vi "CloseDevice.vi"(8 "错误输入（无错误）":errorcluster, 11 "DevIndex":i32) -> (0 "错误输出":errorcluster, 3 "DevIndex Output":i32)   [LabVIEW 2018]
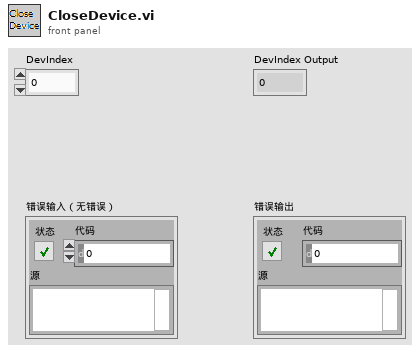
[diagram p1: front panel]
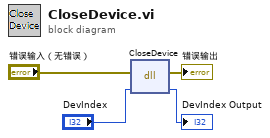
[diagram p0: block diagram]
diagram:
  n1 = dll-call lib="PTH2@abs H科研项目仅一项目程序32位usb-1000.dll" fn="CloseDevice"(error in="错误输入（无错误）", "DevIndex"="DevIndex") -> (error out=→"错误输出":errorcluster, "DevIndex"=→"DevIndex Output":i32)  [unwired: 3 in, 1 out]
